vi "GUI_HPD_BeamPointing.vi"() -> ()   [LabVIEW 2013]
uses:
  shared programs/GUI_Template/GUI_master/tcp_new_data_event.ctl
  shared programs/GUI_Template/GUI_master/tcp new data cluster.ctl
  <vilib>/vision/Image Controls.llb/IMAQ Image.ctl
panel:
  in  "Enable Correction":bool
  in  "FWHMy::1":dbl=0.001 caption="FWHMy" min=0.0 max=999999.0 format="%_4f"
  in  "BP settings":T1={"Max offset (pix)"=20.0, "max allowed counts"=4000.0, "min allowed counts"=200.0, "max allowed FWHM"=100.0, "min allowed FWHM"=0.0}
  in  "FWHMx::1":dbl=0.001 caption="FWHMx" min=0.0 max=999999.0 format="%_4f"
  out "FWHMx in range?":bool
  out "Max counts in range?":bool
  in  "MaxCounts::1":dbl=0.001 caption="MaxCounts" min=0.0 max=999999999.0 format="%_4f"
  in  "relativeMove.Axis 2neg::2":bool caption="Right"
  in  "relativeMove.Axis 2pos::2":bool caption="Left"
  in  "relativeMove.Axis 3pos::2":bool caption="Down"
  in  "relativeMove.Axis 3neg::2":bool caption="relativemove.Axis 3neg::6"
  in  "GUIdevice 2":string="BELLA_ESP_2"
  in  "Target.X::1":dbl=0.001 caption="target x" min=0.0 max=2000.0 format="%_4f"
  in  "Target.Y::1":dbl=0.001 caption="target y" min=0.0 max=2000.0 format="%_4f"
  in  "stop":bool
  in  "trigger::1":bool caption="Trigger"
  in  "gain::1":dbl=0.001 caption="gain" min=0.0 max=12.0 format="%_4f"
  in  "centroidy::1":dbl=0.001 caption="centroid y" min=0.0 max=0.0 format="%_4f"
  in  "centroidx::1":dbl=0.001 caption="centroid x" min=0.0 max=0.0 format="%_4f"
  in  "exposure::1":dbl=0.001 caption="exposure" min=3.8e-05 max=1.0 format="%_4p"
  out "image::1":T2(plugin-control) caption="HPD_CCD Cam"
  in  "GUIdevice 1":string="HPD_CCD"
  out "tcp data event":T3
  out "error IO 2":errorcluster
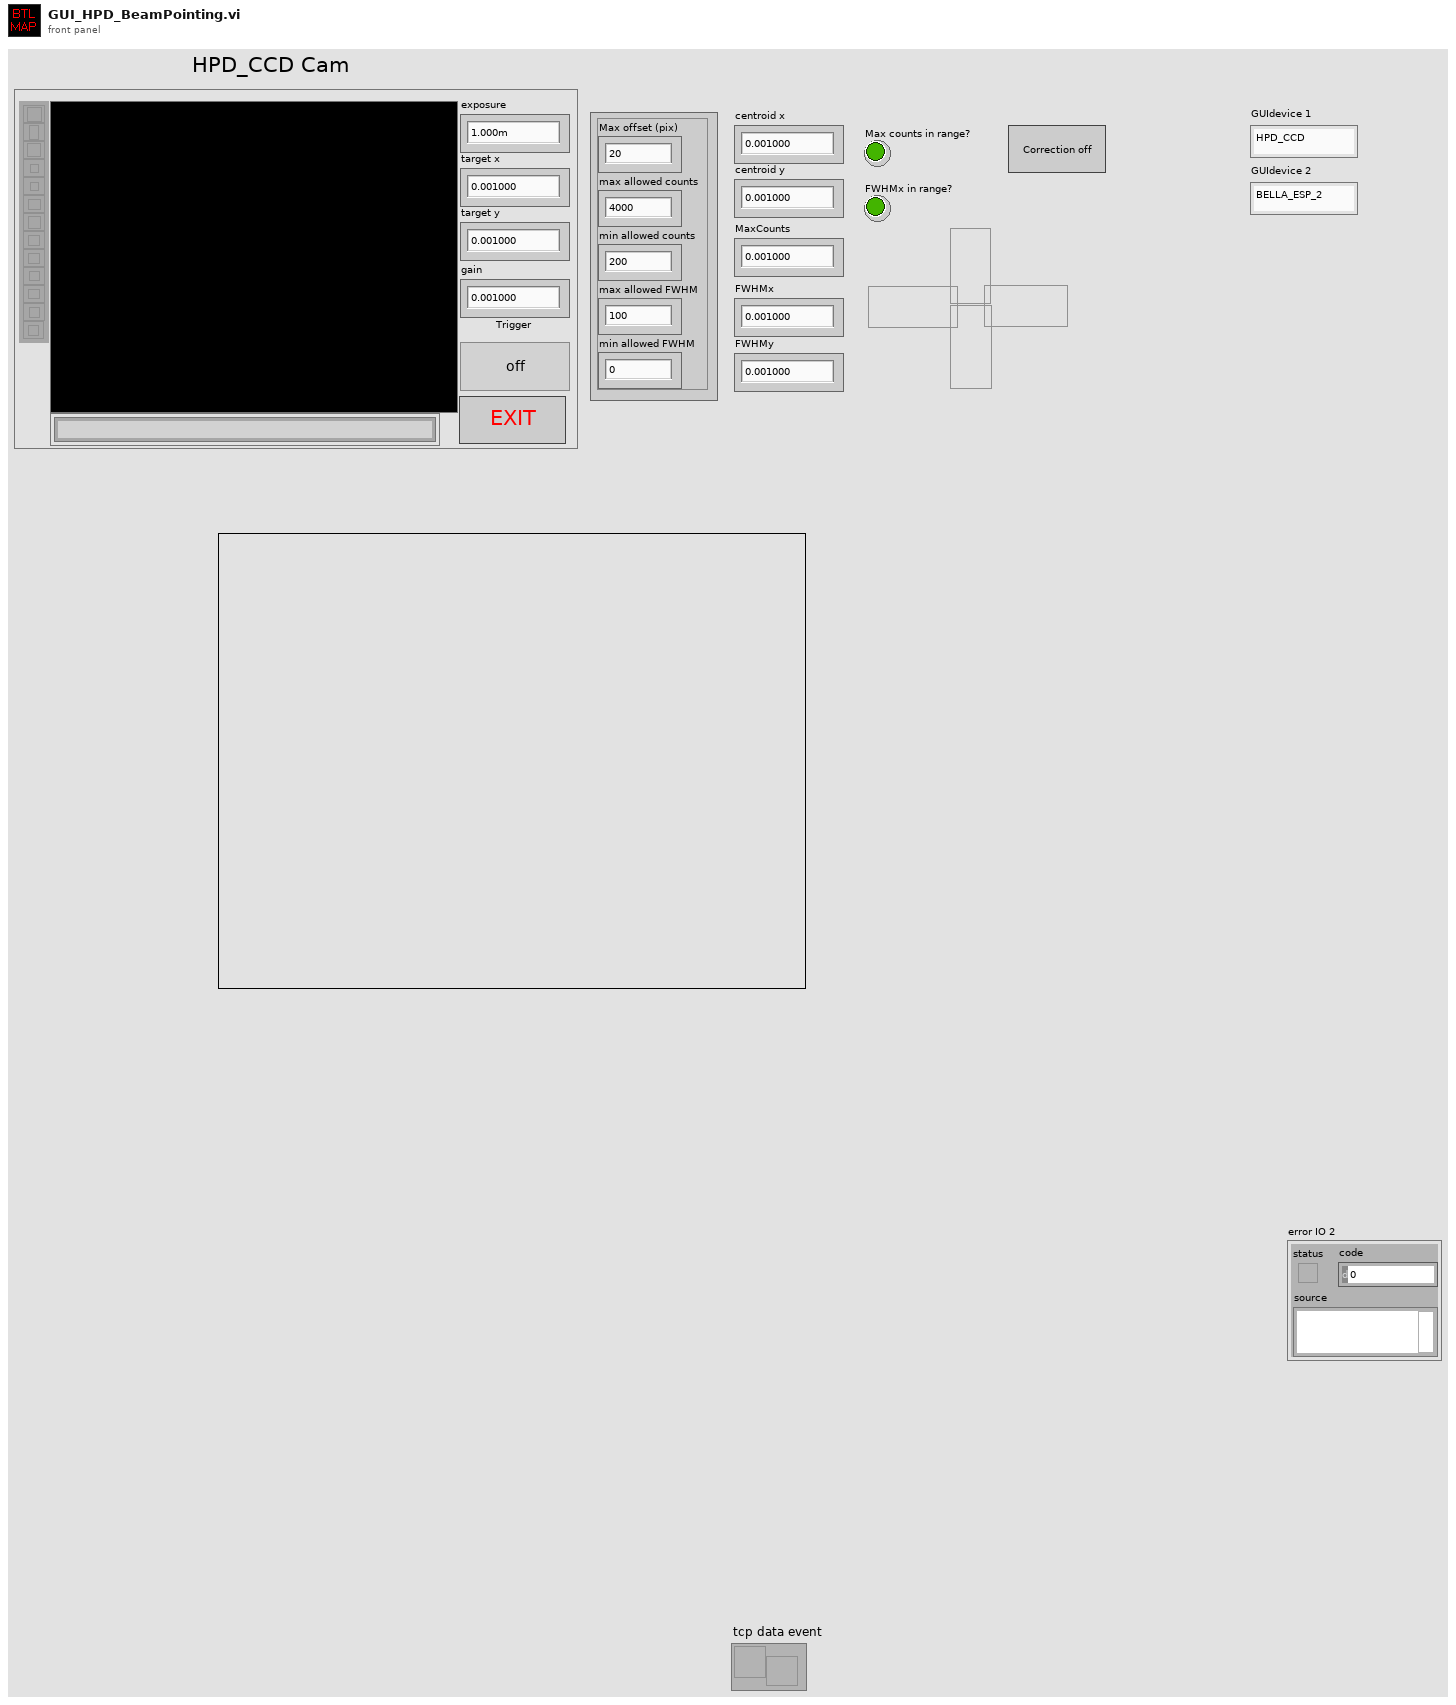
[diagram p1: front panel]
types:
  T1 = cluster{"Max offset (pix)":dbl, "max allowed counts":dbl, "min allowed counts":dbl, "max allowed FWHM":dbl, "min allowed FWHM":dbl}
  T2 = typedef "IMAQ Image.ctl" = refnum<image>
  T3 = typedef "tcp_new_data_event.ctl" = refnum<user-event>
  T4 = typedef "tcp new data cluster.ctl" = cluster{"EventEnum":enum16{"new data", "connection status update"}, "Device name":string}
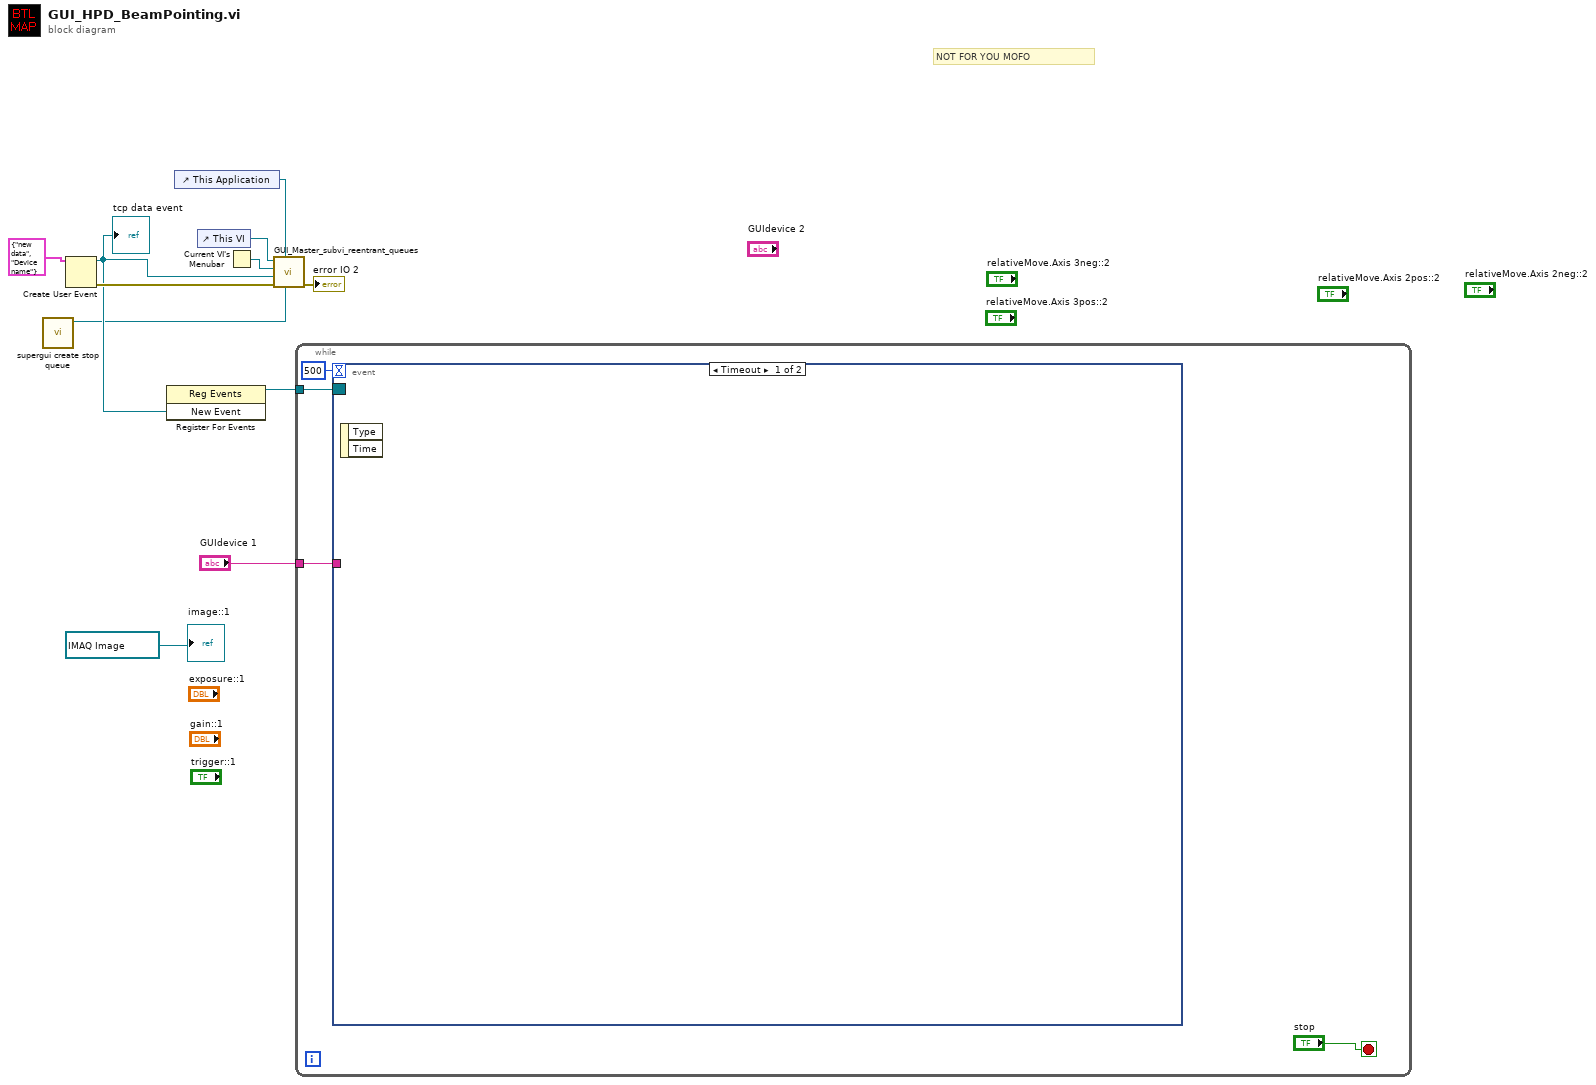
[diagram p0: block diagram]
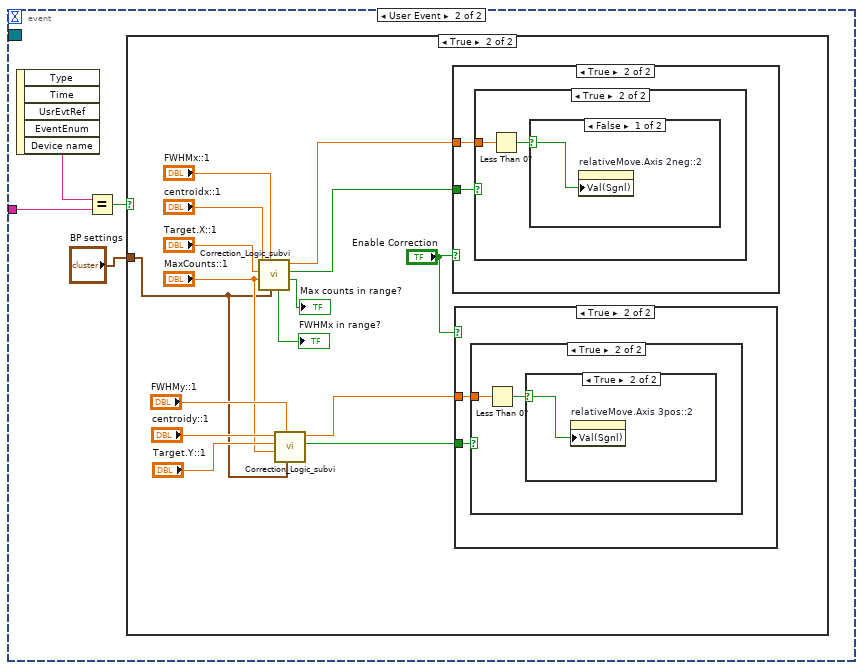
[diagram p2: hidden frame]
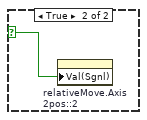
[diagram p6: hidden frame]
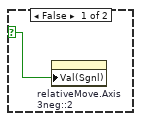
[diagram p9: hidden frame]
diagram:
  # "NOT FOR YOU MOFO"
  n1 = call "supergui create stop queue.vi"() -> ("STOP Queue out"=w1:refnum<queue>)  [unwired: 11 in]
  n2 = Create User Event(user event datatype=T4 {"EventEnum"=enum."new data", "Device name"="Device name"} ("New Event")) -> (user event=w6:refnum<user-event>, error out=w7:errorcluster)  [unwired: 1 in]
  "tcp data event" <- w6
  n3 = register-events(w6) -> (reference out=w4:refnum<event-registration>)  [unwired: 2 in, 1 out]
  n4 = control-ref of="This Application"() -> (w2:refnum<vi>)
  n5 = control-ref of="This VI"() -> (w10:refnum<vi>)
  n6 = Current VI's Menubar() -> (w9:refnum<k9>)
  n7 = call "GUI_Master_subvi_reentrant_queues.vi"("STOP Queue in"=w1, "This Application"=w2, "error in (no error)"=w7, "tcp data event"=w6, "Caller menu reference"=w9, "Caller VI ref"=w10) -> ("error out"=→"error IO 2":errorcluster)  [unwired: 5 in]
  n8 = while {
    tunnel: w4 -> [w14]
    tunnel: "GUIdevice 1" -> [w12]
    stop <- "stop" stop-if-true
    n9 = event shown="[0] Timeout" {
      selector: w14 -> [_ _]
      dyn-events: _ -> [_ _]
      timeout: 500 -> [_ _]
      tunnel: w12 -> [_ w17]
      event Timeout {
        n10 = event-data() -> ()  [unwired: 1 in, 2 out]
      }
      event User Event {
        n11 = event-data() -> ("Device name"=w18:string)  [unwired: 1 in, 4 out]
        n12 = Equal?(x=w18, y=w17) -> (x = y?=w19:bool)
        n13 = case shown="True" w19 {
          tunnel: "BP settings" -> [_ w21]
          frame False {
          }
          frame True {
            n14 = call "Correction_Logic_subvi.vi"("Cluster"=w21, "FWHMx::1"="FWHMx::1", "MaxCounts::1"="MaxCounts::1", "Target.X::1"="Target.X::1", "centroidx::1"="centroidx::1") -> ("Max counts in range?"=→"Max counts in range?":bool, "Correction will be performed"=w31:bool, "offset"=w32:dbl, "FWHMx in range?"=→"FWHMx in range?":bool)  [unwired: 3 in]
            n15 = call "Correction_Logic_subvi.vi"("Cluster"=w21, "FWHMx::1"="FWHMy::1", "MaxCounts::1"="MaxCounts::1", "Target.X::1"="Target.Y::1", "centroidx::1"="centroidy::1") -> ("Correction will be performed"=w27:bool, "offset"=w26:dbl)  [unwired: 3 in, 2 out]
            n16 = case shown="True" "Enable Correction" {
              tunnel: w32 -> [_ w36]
              tunnel: w31 -> [_ w35]
              frame False {
              }
              frame True {
                n17 = case shown="True" w35 {
                  tunnel: w36 -> [_ w38]
                  frame False {
                  }
                  frame True {
                    n18 = Less Than 0?(x=w38) -> (x < 0?=w37:bool)
                    n19 = case shown="False" w37 {
                      selector: w37 -> [w39 w40]
                      frame False {
                        n20 = property on="relativeMove.Axis 2neg::2" class="Bool (strict)"("Val(Sgnl)"=w39) -> ()  [unwired: 2 in, 2 out]
                      }
                      frame True {
                        n21 = property on="relativeMove.Axis 2pos::2" class="Bool (strict)"("Val(Sgnl)"=w40) -> ()  [unwired: 2 in, 2 out]
                      }
                    }
                  }
                }
              }
            }
            n22 = case shown="True" "Enable Correction" {
              tunnel: w27 -> [_ w42]
              tunnel: w26 -> [_ w41]
              frame False {
              }
              frame True {
                n23 = case shown="True" w42 {
                  tunnel: w41 -> [_ w44]
                  frame False {
                  }
                  frame True {
                    n24 = Less Than 0?(x=w44) -> (x < 0?=w43:bool)
                    n25 = case shown="True" w43 {
                      selector: w43 -> [w45 w46]
                      frame False {
                        n26 = property on="relativeMove.Axis 3neg::2" class="Bool (strict)"("Val(Sgnl)"=w45) -> ()  [unwired: 2 in, 2 out]
                      }
                      frame True {
                        n27 = property on="relativeMove.Axis 3pos::2" class="Bool (strict)"("Val(Sgnl)"=w46) -> ()  [unwired: 2 in, 2 out]
                      }
                    }
                  }
                }
              }
            }
          }
        }
      }
    }
  }
  "image::1" <- T2 refnum ("image::1")
